vi "volumeStartCommand.vi"(10 "volume number":i32, 11 "scan specification":T2={"z resolution (pixels)"=1000, "iterations per pixel"=28, "iterations per z-scan (=zres*iterperpixel)"=50, "x resolution (pixels)"=100, "y resolution (pixels)"=80, "number of z-lines per volume"=30, "number of repetitions (volumes)"=5, "Pockels cell voltage (bits)"=-1, "Vx center (bits)"=0, "Vy center (bits)"=0, "Vx amplitude (bits)"=40, "Vy amplitude (bits)"=0, "lines to delay between scan start and output"=1, "LSB has acquire control"=FALSE, "Pockels cell bleach voltage"=0}) -> (3 "scan info":T1)   [LabVIEW 2010]
uses:
  scan_specification_tagResonant.ctl
  scan_command.ctl
  scan message.ctl
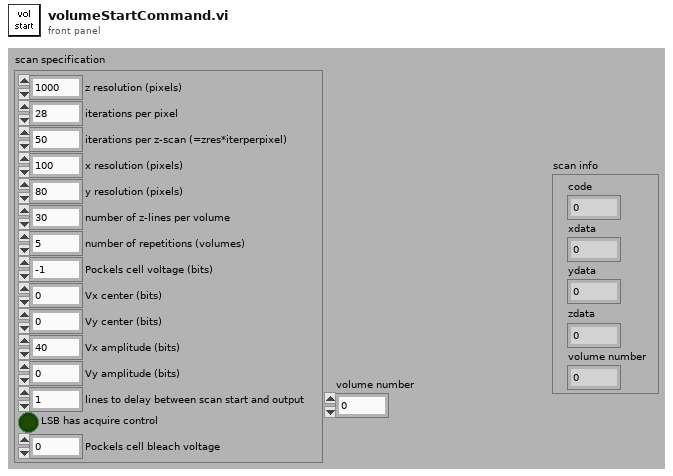
[diagram p1: front panel]
types:
  T1 = typedef "scan_command.ctl" = cluster{"code":i32, "xdata":i32, "ydata":i32, "zdata":i32, "volume number":i32}
  T2 = typedef "scan_specification_tagResonant.ctl" = cluster{"z resolution (pixels)":u16, "iterations per pixel":u16, "iterations per z-scan (=zres*iterperpixel)":u16, "x resolution (pixels)":u16, "y resolution (pixels)":u16, "number of z-lines per volume":u16, "number of repetitions (volumes)":i32, "Pockels cell voltage (bits)":i16, "Vx center (bits)":i16, "Vy center (bits)":i16, "Vx amplitude (bits)":i16, "Vy amplitude (bits)":i16, "lines to delay between scan start and output":u16, "LSB has acquire control":bool, "Pockels cell bleach voltage":i16}
  T3 = typedef "scan message.ctl" = enum8{"NONE", "VOLUME START", "LINE START", "LINE START TRACKING", "XKALMAN", "YKALMAN", "ZKALMAN"}
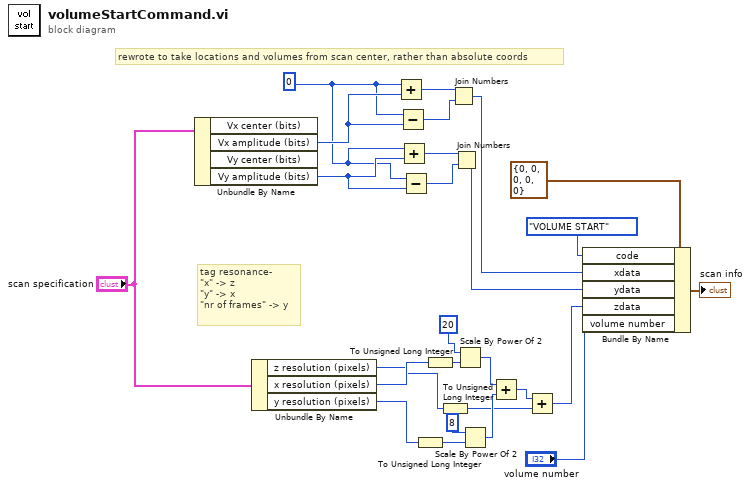
[diagram p0: block diagram]
diagram:
  w1 = i16 0 ("x")
  # "rewrote to take locations and volumes from scan center, rather than absolute coords"
  # "tag resonance-\n\"x\" -> z\n\"y\" -> x\n\"nr of frames\" -> y"
  n1 = Unbundle By Name("scan specification") -> ("Vx amplitude (bits)"=w7:i16, "Vy amplitude (bits)"=w3:i16)  [unwired: 2 out]
  n2 = Unbundle By Name("scan specification") -> ("z resolution (pixels)"=w13:u16, "x resolution (pixels)"=w15:u16, "y resolution (pixels)"=w14:u16)
  n3 = Add(x=w1, y=w7) -> (x+y=w18:i16)
  n4 = Subtract(x=w1, y=w7) -> (x-y=w6:i16)
  n5 = Add(x=w1, y=w3) -> (x+y=w5:i16)
  n6 = Subtract(x=w1, y=w3) -> (x-y=w4:i16)
  n7 = To Unsigned Long Integer(number=w14) -> (unsigned 32bit integer=w9:u32)
  n8 = To Unsigned Long Integer(number=w15) -> (unsigned 32bit integer=w10:u32)
  n9 = To Unsigned Long Integer(number=w13) -> (unsigned 32bit integer=w8:u32)
  n10 = Join Numbers(hi=w18, lo=w6) -> ((hi.lo)=w17:u32)
  n11 = Join Numbers(hi=w5, lo=w4) -> ((hi.lo)=w2:u32)
  n12 = Scale By Power Of 2(n=u8 20 ("x"), x=w10) -> (x*2^n=w26:u32)
  n13 = Scale By Power Of 2(n=u8 8 ("x"), x=w9) -> (x*2^n=w23:u32)
  n14 = Add(x=w26, y=w23) -> (x+y=w22:u32)
  n15 = Add(x=w22, y=w8) -> (x+y=w21:u32)
  n16 = Bundle By Name(cluster=T1 {"code"=0, "xdata"=0, "ydata"=0, "zdata"=0, "volume number"=0} ("scan info"), "code"=scan_message."VOLUME START" ("Enum"), "xdata"=w17, "ydata"=w2, "zdata"=w21, "volume number"="volume number") -> (→"scan info":T1)
